vi "FGV用法_相機光源FGV.vi"   [LabVIEW 2015]
uses:
  <vilib>/userdefined/High Color/IMAQdx.ctl
types:
  T1 = typedef "Control_Indicator Action(FGV).ctl" = enum16{"Set Data", "Get Data", "Idle"}
  T2 = typedef "Control_Indicator(FGV) #.ctl" = cluster{"相機、光源":cluster{"相機選擇":u8, "光源選擇":u16, "光源亮度":u8}, "Session Out":T3, "Cam#Light#Strength":string}
  T3 = typedef "IMAQdx.ctl" = refnum<k21>
  T4 = typedef "光源通訊_action_control.ctl" = enum16{"initial", "開啟光源", "關閉光源", "close"}
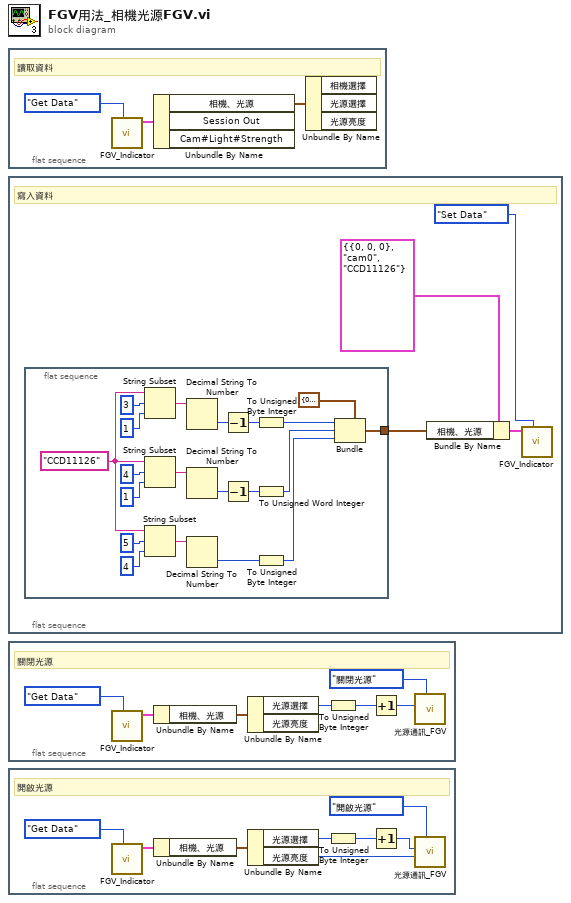
[diagram p0: block diagram]
diagram:
  n1 = flat-sequence {
    frame #0 {
      # "讀取資料"
      n2 = call "FGV_Indicator.vi"("Action"=Control_Indicator_Action(FGV)."Get Data") -> ("Indicator Data Out"=w3:T2)  [unwired: 10 in]
      n3 = Unbundle By Name(w3) -> ("相機、光源"=w1:cluster{"相機選擇":u8, "光源選擇":u16, "光源亮度":u8})  [unwired: 2 out]
      n4 = Unbundle By Name(w1) -> ()  [unwired: 3 out]
    }
  }
  n5 = flat-sequence {
    frame #0 {
      # "寫入資料"
      n6 = flat-sequence {
        tunnel: [w10] -> w4
        frame #0 {
          w8 = "CCD11126" ("Cam#Light#Strength")
          n7 = String Subset(string=w8, offset (0)=3, length (rest)=1 ("length (rest)")) -> (substring=w21:string)
          n8 = String Subset(string=w8, offset (0)=4 ("length (rest)"), length (rest)=1 ("length (rest)")) -> (substring=w26:string)
          n9 = String Subset(string=w8, offset (0)=5 ("length (rest)"), length (rest)=4 ("length (rest)")) -> (substring=w27:string)
          n10 = Decimal String To Number(string=w21) -> (number=w13:i32)  [unwired: 2 in, 1 out]
          n11 = Decimal String To Number(string=w26) -> (number=w15:i32)  [unwired: 2 in, 1 out]
          n12 = Decimal String To Number(string=w27) -> (number=w11:i32)  [unwired: 2 in, 1 out]
          n13 = Decrement(x=w13) -> (x-1=w12:i32)
          n14 = Decrement(x=w15) -> (x-1=w14:i32)
          n15 = To Unsigned Byte Integer(number=w12) -> (unsigned 8bit integer=w18:u8)
          n16 = To Unsigned Word Integer(number=w14) -> (unsigned 16bit integer=w17:u16)
          n17 = To Unsigned Byte Integer(number=w11) -> (unsigned 8bit integer=w16:u8)
          n18 = Bundle(cluster=cluster{"相機選擇":u8, "光源選擇":u16, "光源亮度":u8} {"相機選擇"=0, "光源選擇"=0, "光源亮度"=0} ("相機、光源"), "相機選擇"=w18, "光源選擇"=w17, "光源亮度"=w16) -> (w10:cluster{"相機選擇":u8, "光源選擇":u16, "光源亮度":u8})
        }
      }
      n19 = Bundle By Name(cluster=T2 {"相機、光源"={"相機選擇"=0, "光源選擇"=0, "光源亮度"=0}, "Session Out"="cam0", "Cam#Light#Strength"="CCD11126"} ("Indicator Data In"), "相機、光源"=w4) -> (w5:T2)
      n20 = call "FGV_Indicator.vi"("Action"=Control_Indicator_Action(FGV)."Set Data", "Indicator Data In"=w5) -> ()  [unwired: 9 in, 1 out]
    }
  }
  n21 = flat-sequence {
    frame #0 {
      # "關閉光源"
      n22 = call "FGV_Indicator.vi"("Action"=Control_Indicator_Action(FGV)."Get Data") -> ("Indicator Data Out"=w32:T2)  [unwired: 10 in]
      n23 = Unbundle By Name(w32) -> ("相機、光源"=w31:cluster{"相機選擇":u8, "光源選擇":u16, "光源亮度":u8})
      n24 = Unbundle By Name(w31) -> ("光源選擇"=w30:u16)  [unwired: 1 out]
      n25 = To Unsigned Byte Integer(number=w30) -> (unsigned 8bit integer=w29:u8)
      n26 = Increment(x=w29) -> (x+1=w28:u8)
      n27 = call "光源通訊_FGV.vi"("通訊_action"=光源通訊_action_control."關閉光源", "通道"=w28) -> ()  [unwired: 8 in, 2 out]
    }
  }
  n28 = flat-sequence {
    frame #0 {
      # "開啟光源"
      n29 = call "FGV_Indicator.vi"("Action"=Control_Indicator_Action(FGV)."Get Data") -> ("Indicator Data Out"=w40:T2)  [unwired: 10 in]
      n30 = Unbundle By Name(w40) -> ("相機、光源"=w39:cluster{"相機選擇":u8, "光源選擇":u16, "光源亮度":u8})
      n31 = Unbundle By Name(w39) -> ("光源選擇"=w37:u16, "光源亮度"=w38:u8)
      n32 = To Unsigned Byte Integer(number=w37) -> (unsigned 8bit integer=w36:u8)
      n33 = Increment(x=w36) -> (x+1=w35:u8)
      n34 = call "光源通訊_FGV.vi"("通訊_action"=光源通訊_action_control."開啟光源", "亮度"=w38, "通道"=w35) -> ()  [unwired: 7 in, 2 out]
    }
  }
